vi "Read value type.vi"(8 "error in (no error)":errorcluster, 11 "rqcBob in":refnum<class "rqcBob.lvclass">) -> (0 "error out":errorcluster, 2 "RndGen.Value Type":T1=enum."constant", 3 "rqcBob out":refnum<class "rqcBob.lvclass">)   [LabVIEW 2018, in "rqcBob.lvclass"]
uses:
  rqcBob.lvclass
  Shared/Shared FPGA Lib/Shared Logic/Custom Controls/rqc Random Generator.value type.ctl
  rqcBob.lvclass/rqcBob.ctl
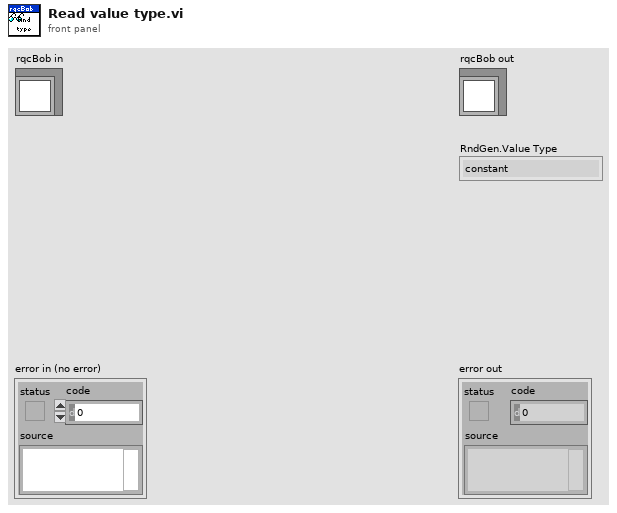
[diagram p1: front panel]
types:
  T1 = typedef "rqc Random Generator.value type.ctl" = enum16{"random value", "constant"}
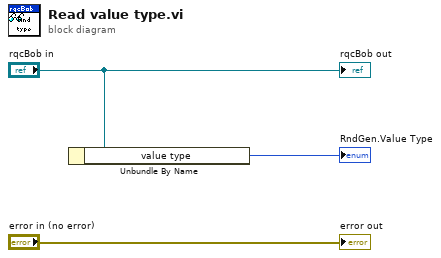
[diagram p0: block diagram]
diagram:
  n1 = Unbundle By Name("rqcBob in") -> ("value type"=→"RndGen.Value Type":T1)
  "error out" <- "error in (no error)"
  "rqcBob out" <- "rqcBob in"
